vi "calcForceMeasured.vi"(8 "error in (no error)":errorcluster, 11 "ForceSensor in":refnum<class "ForceSensor.lvclass">) -> (0 "error out":errorcluster, 3 "ForceSensor out":refnum<class "ForceSensor.lvclass">)   [LabVIEW 2013, in "ForceSensor.lvclass"]
uses:
  ForceSensor.lvclass
  ForceSensor.lvclass/ForceSensor.ctl
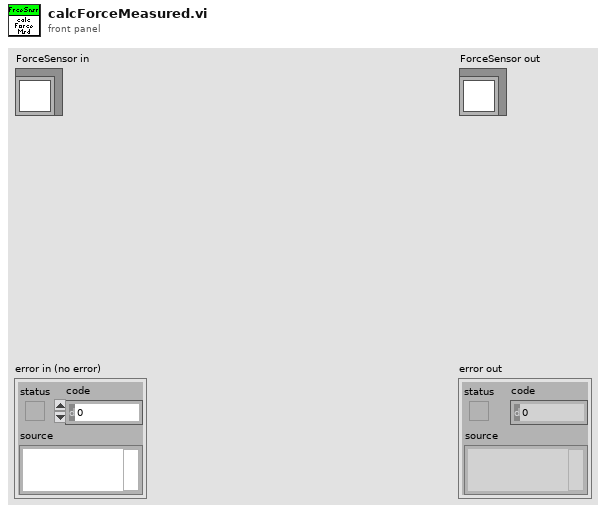
[diagram p1: front panel]
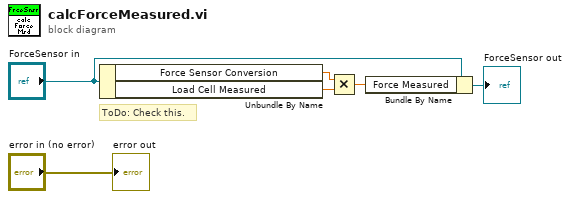
[diagram p0: block diagram]
diagram:
  # "ToDo: Check this."
  n1 = Unbundle By Name("ForceSensor in") -> ("Force Sensor Conversion"=w2:dbl[unit], "Load Cell Measured"=w3:dbl[unit])
  n2 = Multiply(x=w2, y=w3) -> (x*y=w1:dbl[unit])
  n3 = Bundle By Name(cluster="ForceSensor in", "Force Measured"=w1) -> (→"ForceSensor out":refnum<class "ForceSensor.lvclass">)
  "error out" <- "error in (no error)"
